vi "DER_setGenerationMode_subTest.vi"(7 "Test Result in":T2=enum."Success", 8 "error in":errorcluster, 9 "DeviceID":T1, 10 "MicrogridID":u8, 11 "Message Enqueuer in":refnum<class "Message Enqueuer.lvclass">) -> (0 "error out":errorcluster, 1 "dup DeviceID":T1, 2 "dup MicrogridID":u8, 3 "Message Enqueuer out":refnum<class "Message Enqueuer.lvclass">, 5 "Test Result out":T2=enum."Success")   [LabVIEW 2018, in "IED Test Framework.lvlib" / "IED Test.lvclass"]
uses:
  IED Test.lvclass
  <vilib>/ActorFramework/Message Enqueuer/Message Enqueuer.lvclass
  Controls/Test Result.ctl
  <vilib>/ORNL/CSEISMIC DDS/CSEISMIC DDS Base/Data Types/Controls/DeviceID.ctl
  <vilib>/ORNL/CSEISMIC DDS/CSEISMIC DDS Base/Data Types/DER_setGenerationMode.ctl
  <vilib>/ORNL/CSEISMIC DDS/CSEISMIC DDS Base/Data Types/Controls/Generation Mode.ctl
  <vilib>/ORNL/CSEISMIC DDS/CSEISMIC DDS Base/CSEISMIC DDS.lvclass/CSEISMIC DDS.ctl
  DER Actor/DER Messages/Write DER setGenerationMode Msg/Write DER setGenerationMode Msg.lvclass/Write DER setGenerationMode Msg.ctl
  <vilib>/ActorFramework/Message Enqueuer/Message Enqueuer.lvclass/Message Enqueuer.ctl
  <vilib>/ORNL/CSEISMIC DDS/CSEISMIC DDS Base/Accessors/Write DDS Reference.vi
  <vilib>/ORNL/CSEISMIC DDS/CSEISMIC DDS Base/Accessors/Read DDS Reference.vi
  <vilib>/ActorFramework/Message Enqueuer/Enqueue.vi
  <vilib>/ORNL/CSEISMIC DDS/DDS Reader/DDS Reader.lvclass
  C:/Program Files (x86)/National Instruments/LabVIEW 2018/vi.lib/ORNL/CSEISMIC DDS/CSEISMIC DDS Base/CSEISMIC DDS.lvclass
  DER Actor/DER Messages/Write DER setGenerationMode Msg/Write DER setGenerationMode Msg.lvclass
  C:/Program Files (x86)/National Instruments/LabVIEW 2018/vi.lib/ActorFramework/Message/Message.lvclass
  <vilib>/ORNL/CSEISMIC DDS/CSEISMIC DDS Base/Error Handler.vi
  <vilib>/ActorFramework/Message Priority Queue/Priority Enqueue.vi
  <vilib>/ORNL/CSEISMIC DDS/CSEISMIC DDS Base/CSEISMIC DDS.lvclass
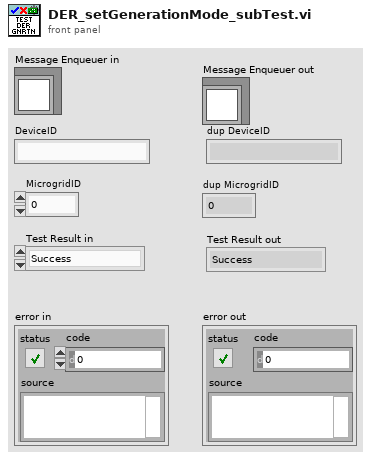
[diagram p1: front panel]
types:
  T1 = typedef "CSEISMIC DDS.lvlib/CSEISMIC DDS.lvclass/DeviceID.ctl" = string
  T2 = typedef "IED Test Framework.lvlib/IED Test.lvclass/Test Result.ctl" = enum16{"Invalid", "Success", "Failure", "Error", "Timeout"}
  T3 = typedef "CSEISMIC DDS.lvlib/CSEISMIC DDS.lvclass/DER_setGenerationMode.ctl" = cluster{"DeviceID":T1, "Mode":T4}
  T4 = typedef "CSEISMIC DDS.lvlib/CSEISMIC DDS.lvclass/Generation Mode.ctl" = enum32{"Invalid", "PQ", "Droop", "PV", "PF", "VF"}
  T5 = typedef "LVDDS_library.lvlib/DDS Sample Info.ctl" = cluster{"DDS_SampleStateKind":enum32{"DDS_INVALID_SAMPLE_STATE", "DDS_READ_SAMPLE_STATE", "DDS_NOT_READ_SAMPLE_STATE"}, "DDS_ViewStateKind":enum32{"DDS_INVALID_SAMPLE_STATE", "DDS_NEW_VIEW_STATE", "DDS_NOT_NEW_VIEW_STATE"}, "DDS_InstanceStateKind":enum32{"DDS_INVALID_STATE", "DDS_ALIVE_INSTANCE_STATE", "DDS_NOT_ALIVE_DISPOSED_INSTANCE_STATE", "", "DDS_NOT_ALIVE_NO_WRITERS_INSTANCE_STATE"}, "sec":i32, "nanosec":u32, "valid_data":bool}
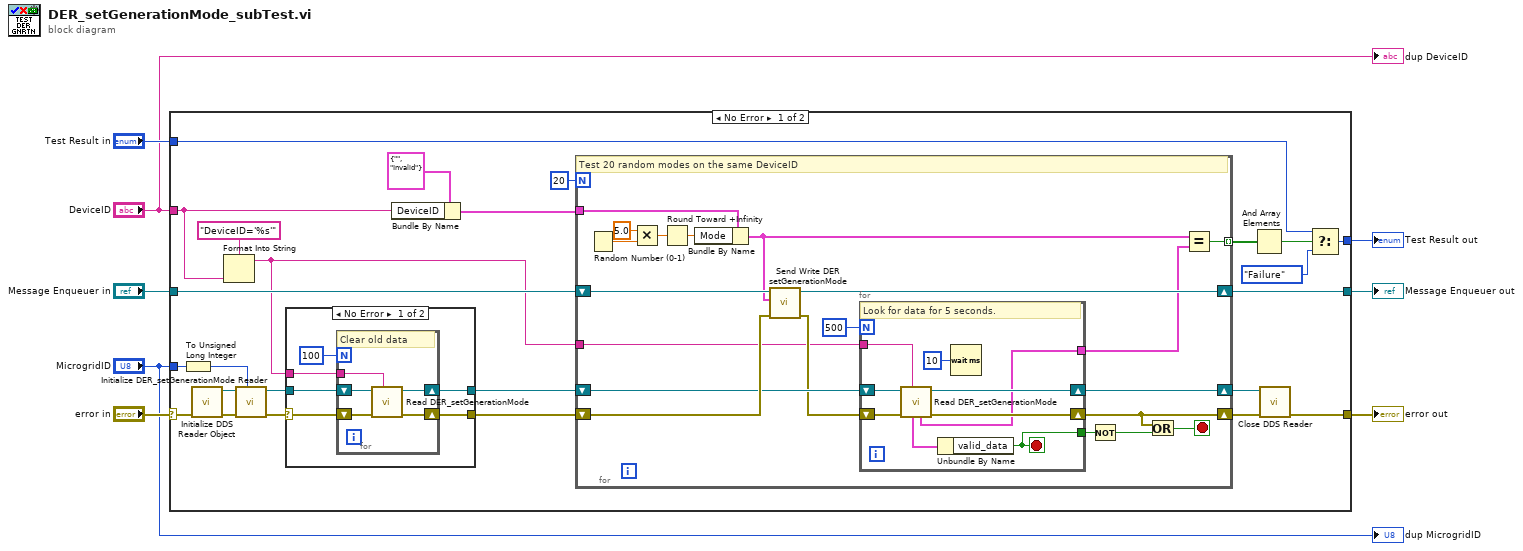
[diagram p0: block diagram]
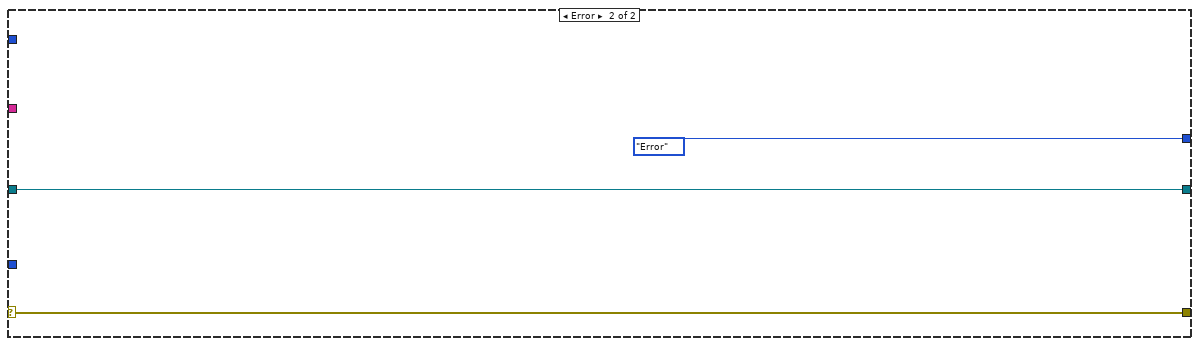
[diagram p3: hidden frame]
diagram:
  n1 = case shown="No Error" "error in" {
    selector: "error in" -> [w22 w78]
    tunnel: "Test Result in" -> [w28 _]
    tunnel: [w27 Test_Result."Error" ("f")] -> w7
    tunnel: "DeviceID" -> [w11 _]
    tunnel: "MicrogridID" -> [w18 _]
    tunnel: [w13 w78] -> w6
    tunnel: [w26 w77] -> w5
    tunnel: "Message Enqueuer in" -> [w25 w77]
    frame No Error {
      n2 = To Unsigned Long Integer(number=w18) -> (unsigned 32bit integer=w16:u32)
      n3 = call <vilib>:"Initialize DDS Reader Object.vi"("error in"=w22) -> ("error out"=w21:errorcluster, "DDS Reader out"=w19:refnum<class "DDS Reader.lvclass">)  [unwired: 9 in]
      n4 = Format Into String(format string="DeviceID='%s'", w11) -> (resulting string=w9:string)  [unwired: 2 in, 1 out]
      n5 = call <vilib>:"Initialize DER_setGenerationMode Reader.vi"("MicrogridID"=w16, "error in"=w21, "DDS Reader in"=w19) -> ("error out"=w20:errorcluster, "DDS Reader out"=w17:refnum<class "DDS Reader.lvclass">)  [unwired: 7 in]
      n6 = case shown="No Error" w20 {
        selector: w20 -> [w68 w75]
        tunnel: [w67 w75] -> w30
        tunnel: w17 -> [w66 w74]
        tunnel: [w65 w74] -> w24
        tunnel: w9 -> [w63 _]
        frame No Error {
          n7 = for {
            N: 100 -> [_]
            shift-right: [w73] -> w67
            shift-left: w68 -> [w70]
            shift-right: [w71] -> w65
            shift-left: w66 -> [w72]
            tunnel: w63 -> [w69]
            # "Clear old data"
            n8 = call <vilib>:"Read DER_setGenerationMode.vi"("Query condition"=w69, "error in"=w70, "DDS Reader in"=w72) -> ("error out"=w73:errorcluster, "DDS Reader out"=w71:refnum<class "DDS Reader.lvclass">)  [unwired: 5 in, 2 out]
          }
        }
        frame Error {
        }
      }
      n9 = Bundle By Name(cluster=T3 {"DeviceID"="", "Mode"=enum."Invalid"} ("DER_setGenerationMode"), "DeviceID"=w11) -> (w10:T3)
      n10 = for {
        N: 20 -> [_]
        tunnel: w10 -> [w37]
        tunnel: [w48] -> w33 mode=indexing
        shift-right: [w43] -> w15
        shift-left: w30 -> [w52]
        shift-right: [w45] -> w14
        shift-left: w24 -> [w46]
        shift-right: [w53] -> w26
        shift-left: w25 -> [w47]
        tunnel: w9 -> [w34]
        stop <- w41 stop-if-true
        # "Test 20 random modes on the same DeviceID"
        n11 = Random Number (0-1)() -> (number: 0 to 1=w51:dbl)
        n12 = Multiply(x=5.0, y=w51) -> (x*y=w49:dbl)
        n13 = Round Toward +Infinity(x=w49) -> (ceil(x): smallest int >= x=w35:dbl)
        n14 = Bundle By Name(cluster=w37, "Mode"=w35) -> (w36:T3)
        n15 = call "Send Write DER setGenerationMode.vi"("error in (no error)"=w52, "DER_setGenerationMode"=w36, "Message Enqueuer"=w47) -> ("error out"=w44:errorcluster, "Message Enqueuer out"=w53:refnum<class "Message Enqueuer.lvclass">)  [unwired: 7 in]
        n16 = for {
          N: 500 -> [_]
          tunnel: [w55] -> w40
          shift-right: [w58] -> w43
          shift-left: w44 -> [w61]
          shift-right: [w59] -> w45
          shift-left: w46 -> [w60]
          tunnel: [w56] -> w42
          tunnel: w34 -> [w54]
          stop <- w56 stop-if-true
          # "Look for data for 5 seconds."
          n17 = call <vilib>:"Read DER_setGenerationMode.vi"("Query condition"=w54, "error in"=w61, "DDS Reader in"=w60) -> ("error out"=w58:errorcluster, "DDS Reader out"=w59:refnum<class "DDS Reader.lvclass">, "data"=w55:T3, "DDS Sample Info"=w57:T5)  [unwired: 5 in]
          n18 = Unbundle By Name(w57) -> ("valid_data"=w56:bool)
          n19 = Wait (ms)(milliseconds to wait=u32 10) -> ()  [unwired: 1 out]
        }
        n20 = Not(x=w42) -> (.not. x?=w38:bool)
        n21 = Or(x=w43, y=w38) -> (x .or. y?=w41:bool)
        n22 = Equal?(x=w36, y=w40) -> (x = y?=w48:bool)
      }
      n23 = And Array Elements(Boolean array=w33) -> (logical AND=w32:bool)
      n24 = call <vilib>:"Close DDS Reader.vi"("error in"=w15, "DDS Reader in"=w14) -> ("error out"=w13:errorcluster)  [unwired: 9 in]
      n25 = Select(t=w28, s=w32, f=Test_Result."Failure") -> (s? t:f=w27:T2)
    }
    frame Error {
    }
  }
  "Test Result out" <- w7
  "error out" <- w6
  "Message Enqueuer out" <- w5
  "dup DeviceID" <- "DeviceID"
  "dup MicrogridID" <- "MicrogridID"
